vi "Get Diameter from Voltage.vi"(8 "error in":errorcluster, 10 "Vin":dbl, 11 "DMA in":refnum<class "DMA.lvclass">) -> (0 "error out":errorcluster, 2 "Dout":dbl, 3 "DMA out":refnum<class "DMA.lvclass">)   [LabVIEW 2014, in "DMA.lvclass"]
doc: "Retrieve the calculated diameter from a given voltage. This is done by setting the theoretical electrical mobility calculated from the voltage to the particle mobility (Zv = Zd). The diameter returned will also be a function of the ambient flow properties. This includes temperature, pressure and flow rates."
uses:
  DMA.lvclass
  DMA.lvclass/DMA.ctl
  Dz from V.vi
  <vilib>/gmath/zero.llb/Ridders Zero Finder (VI).vi
  <vilib>/gmath/NI_Gmath.lvlib
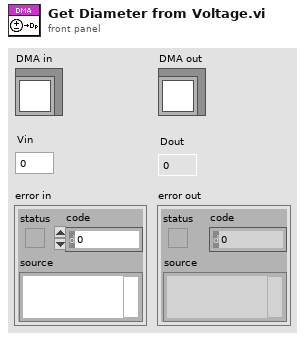
[diagram p1: front panel]
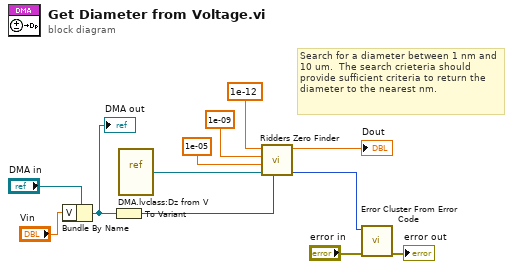
[diagram p0: block diagram]
diagram:
  # "Search for a diameter between 1 nm and 10 um.  The search crieteria should provide sufficient criteria to return the diameter to the nearest nm."
  n1 = Bundle By Name(cluster="DMA in", "V"="Vin") -> (w1:refnum<class "DMA.lvclass">)
  "DMA out" <- w1
  n2 = To Variant(anything=w1) -> (Variant=w9:variant)
  n3 = vi-ref "DMA.lvclass:Dz from V.vi"() -> (w12:refnum<vi>)
  n4 = call-poly <vilib>:"Ridders Zero Finder.vi"("data"=w9, "f(x)"=w12, "end"=1e-05, "start"=1e-09, "accuracy"=1e-12) -> ("error"=w4:i32, "zero"=→"Dout":dbl)  [unwired: 3 in, 2 out]
  n5 = call <vilib>:"Error Cluster From Error Code.vi"("error in (no error)"="error in", "error code (0)"=w4) -> ("error out"=→"error out":errorcluster)  [unwired: 7 in]
